vi "Callback - Get Plottable Names.vi"(8 "error in (no error)":errorcluster, 11 "BluePlotHandleDemo in":refnum<class "BluePlotHandleDemo.lvclass">) -> (0 "error out":errorcluster, 2 "Plottable Names":string[](array[string]), 3 "BluePlotHandleDemo out":refnum<class "BluePlotHandleDemo.lvclass">)   [LabVIEW 2021, in "BluePlotDemo.lvlib" / "BluePlotHandleDemo.lvclass"]
uses:
  BluePlotHandleDemo.lvclass
  BluePlotHandleDemo.lvclass/BluePlotHandleDemo.ctl
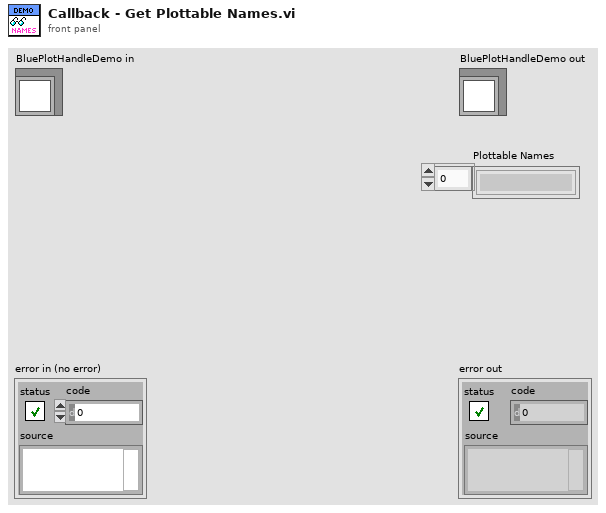
[diagram p1: front panel]
types:
  T1 = typedef "BluePlotDemo.lvlib/Demo Names.ctl" = enum16{"Sine Wave", "Triangle Wave", "Sawtooth Wave", "Square Wave", "Uniform Noise", "Periodic Noise", "White Noise"}
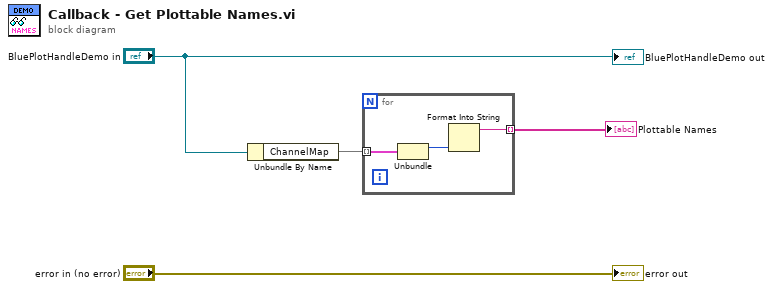
[diagram p0: block diagram]
diagram:
  n1 = Unbundle By Name("BluePlotHandleDemo in") -> ("ChannelMap"=w3:map{T1, refnum<data-value>})
  n2 = for {
    tunnel: w3 -> [w6] mode=indexing
    tunnel: [w7] -> w2 mode=indexing
    n3 = Unbundle(w6) -> ("channel"=w5:T1)  [unwired: 1 out]
    n4 = Format Into String(w5) -> (resulting string=w7:string)  [unwired: 3 in, 1 out]
  }
  "Plottable Names" <- w2
  "error out" <- "error in (no error)"
  "BluePlotHandleDemo out" <- "BluePlotHandleDemo in"
